vi "Read Avg Finger Speed.vi"(0 "Tip Velocity Module":sgl[](array[numeric]), 1 "Array v istantanee  IN":sgl[][](array[numeric]), 2 "Array vel medie IN":sgl[][](array[numeric]), 3 "Error In":errorcluster) -> (5 "Array vel medie OUT":sgl[][](array[numeric]), 6 "Velocità medie finali":sgl[](array[numeric]), 7 "Array v istantanee OUT":sgl[][](array[numeric]), 8 "velocità medie istantanee out":dbl[](array[numeric]), 9 "Error Out":errorcluster)   [LabVIEW 2014]
uses:
  <vilib>/Analysis/baseanly.llb/Mean (DBL).vi
  <vilib>/Analysis/NI_AALBase.lvlib
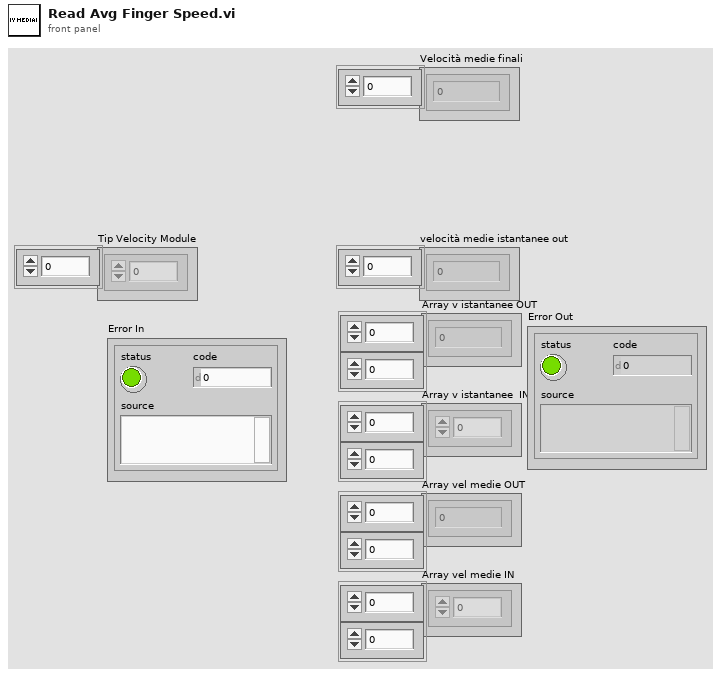
[diagram p1: front panel]
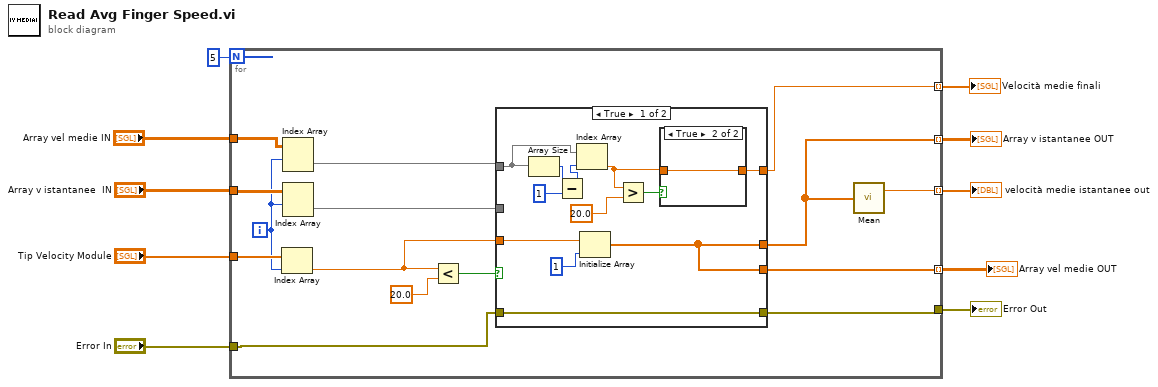
[diagram p0: block diagram]
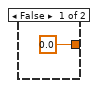
[diagram p2: hidden frame]
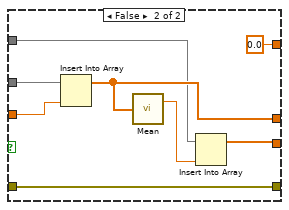
[diagram p3: hidden frame]
diagram:
  n1 = for {
    N: 5 -> [_]
    tunnel: [w23] -> w9 mode=indexing
    tunnel: [w22] -> w7 mode=indexing
    tunnel: "Tip Velocity Module" -> [w21]
    tunnel: "Array v istantanee  IN" -> [w20]
    tunnel: [w18] -> w4
    tunnel: "Error In" -> [w17]
    tunnel: "Array vel medie IN" -> [w13]
    tunnel: [w15] -> w3 mode=indexing
    tunnel: [w11] -> w1 mode=indexing
    i -> [w14]
    n2 = Index Array(array=w21, index=w14) -> (element=w16:sgl)
    n3 = Index Array(array=w13, index (row)=w14) -> (element=w12:sgl[])  [unwired: 1 in]
    n4 = Index Array(array=w20, index (row)=w14) -> (element=w19:sgl[])  [unwired: 1 in]
    n5 = Less?(x=w16, y=sgl 20.0) -> (x < y?=w24:bool)
    n6 = case shown="True" w24 {
      tunnel: [w26 w44] -> w22
      tunnel: w16 -> [w33 w46]
      tunnel: w19 -> [_ w47]
      tunnel: [w36 w45] -> w18
      tunnel: w17 -> [w36 w45]
      tunnel: w12 -> [w31 w41]
      tunnel: [w26 w43] -> w15
      tunnel: [w32 sgl 0.0 ("sqrt(x)")] -> w11
      frame True {
        n7 = Array Size(array=w31) -> (size(s)=w29:i32)
        n8 = Subtract(x=w29, y=1) -> (x-y=w28:i32)
        n9 = Index Array(array=w31, index=w28) -> (element=w30:sgl)
        n10 = Initialize Array(w33, 1 ("dimension size")) -> (w26:sgl[])
        n11 = Greater?(x=w30, y=sgl 20.0) -> (0:w34:bool)
        n12 = case shown="True" w34 {
          tunnel: w30 -> [_ w39]
          tunnel: [sgl 0.0 ("sqrt(x)") w39] -> w32
          frame False {
          }
          frame True {
          }
        }
      }
      frame False {
        n13 = Insert Into Array(array=w47, new element=w46) -> (w44:sgl[])  [unwired: 1 in]
        n14 = call-poly <vilib>:"Mean.vi"("X"=w44) -> ("mean"=w40:dbl)  [unwired: 1 out]
        n15 = Insert Into Array(array=w41, new element=w40) -> (w43:sgl[])  [unwired: 1 in]
      }
    }
    n16 = call-poly <vilib>:"Mean.vi"("X"=w22) -> ("mean"=w23:dbl)  [unwired: 1 out]
  }
  "velocità medie istantanee out" <- w9
  "Array v istantanee OUT" <- w7
  "Error Out" <- w4
  "Array vel medie OUT" <- w3
  "Velocità medie finali" <- w1
